vi "publish -- set frequency.vi"(7 "publisher action":T1, 10 "freq IN (Hz)":dbl=1000.0) -> (2 "freq out (Hz)":dbl=1000.0)   [LabVIEW 2021]
uses:
  publisher action.ctl
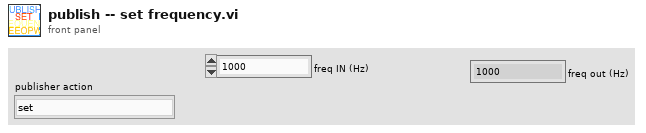
[diagram p1: front panel]
types:
  T1 = typedef "publisher action.ctl" = enum16{"set", "get", "init", "check"}
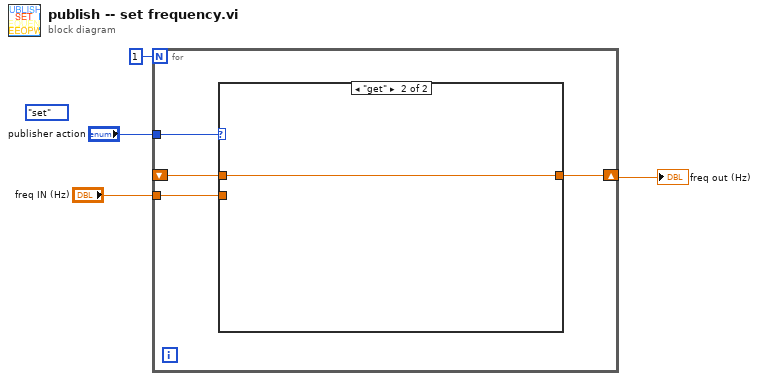
[diagram p0: block diagram]
diagram:
  (unwired) publisher_action."set" ("publisher action")
  n1 = for {
    N: 1 -> [_]
    tunnel: "publisher action" -> [w8]
    tunnel: "freq IN (Hz)" -> [w6]
    shift-right: [w7] -> w1
    shift-left: _ -> [w5]
    n2 = case shown="\"get\"" w8 {
      tunnel: [w9 w10] -> w7
      tunnel: w6 -> [w9 _]
      tunnel: w5 -> [_ w10]
      frame "set", Default {
      }
      frame "get" {
      }
    }
  }
  "freq out (Hz)" <- w1
